vi "Interface.vi"() -> ()   [LabVIEW 2016, in "Program Interface.lvclass"]
uses:
  Program Interface.lvclass
  Universal Robot/Universal Robot.lvclass
  C:/_Code/Development/UR LabVIEW Interface/Classes/Application Interface/Application Interface.lvclass
  Universal Robot/ProgramControlEvent.ctl
  Program Interface.lvclass/Program Interface.ctl
  Application/Application.lvclass
  Application Interface/Application Interface.lvclass
panel:
  out "loadedProgram":string
  out "programStatus":string
  out "programStatusColor":u32(colorbox)
  in  "play":bool
  in  "pause":bool
  in  "stop":bool
  out "returnStatus":string
  in  "load":bool
  in  "programList":i32(listbox)
  in  "addProgram":string
  in  "add program":bool
  in  "play queue":bool
  in  "programQueue":i32(listbox)
  in  "clear queue":bool
  in  "interface":refnum<class "Program Interface.lvclass">
  in  "robot":refnum<class "Universal Robot.lvclass">
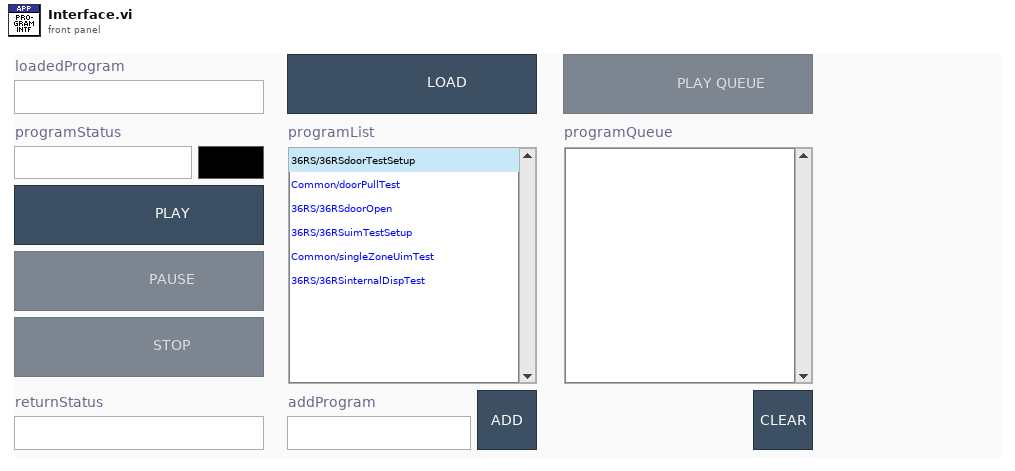
[diagram p1: front panel]
types:
  T1 = typedef "Universal Robot.lvclass/ProgramControlEvent.ctl" = enum16{"Stop", "Pause"}
  T2 = typedef "Application.lvclass/FrontPanelControls.ctl" = cluster{"General Interface":refnum<vi>, "Program Interface":refnum<vi>, "Command Interface":refnum<vi>}
  T3 = typedef "Universal Robot.lvclass/RobotStatus.ctl" = cluster{"Robot Mode":T4, "Operational Mode":T5, "Safety Status":T6, "Remote Control":bool}
  T4 = typedef "Universal Robot.lvclass/RobotMode.ctl" = enum16{"INVALID", "NO_CONTROLLER", "DISCONNECTED", "CONFIRM_SAFETY", "BOOTING", "POWER_OFF", "POWER_ON", "IDLE", "BACKDRIVE", "RUNNING"}
  T5 = typedef "Universal Robot.lvclass/OperationalMode.ctl" = enum16{"NONE", "MANUAL", "AUTOMATIC"}
  T6 = typedef "Universal Robot.lvclass/SafetyStatus.ctl" = enum16{"INVALID", "NORMAL", "REDUCED", "PROTECTIVE_STOP", "RECOVERY", "SAFEGAURD_STOP", "SYSTEM_EMERGENCY_STOP", "ROBOT_EMERGENCY_STOP", "VIOLATION", "FAULT", "AUTOMATIC_MODE_SAFEGAURD_STOP", "SYSTEM_THREE_POSITION_ENABLING_STOP"}
  T7 = typedef "Universal Robot.lvclass/ProgramStatus.ctl" = cluster{"Loaded Program":string, "Valid Program":bool, "Program State":T8, "Running":bool}
  T8 = typedef "Universal Robot.lvclass/ProgramState.ctl" = enum16{"STOPPED", "PLAYING", "PAUSE"}
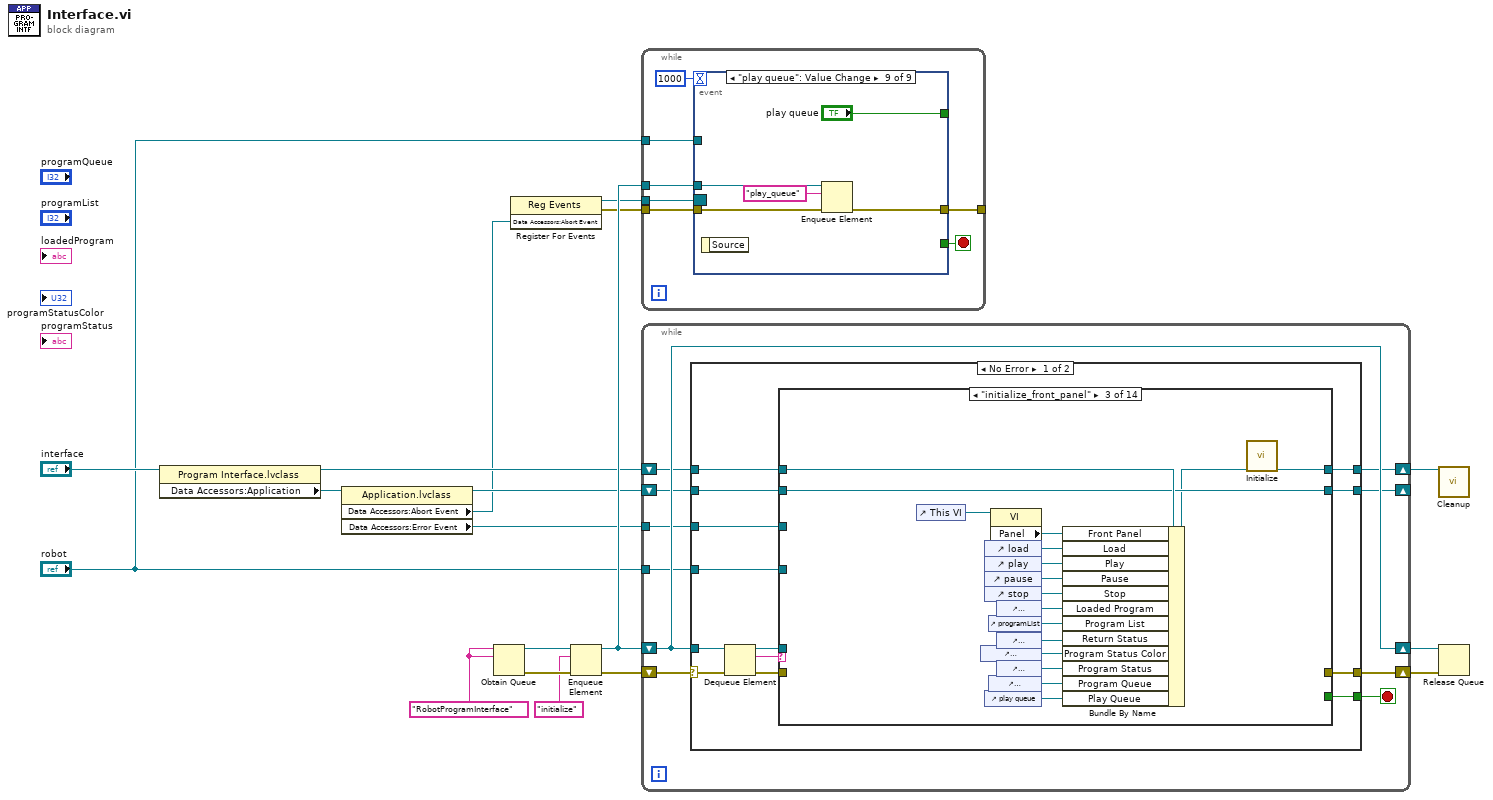
[diagram p0: block diagram]
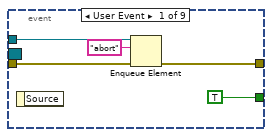
[diagram p2: hidden frame]
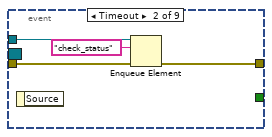
[diagram p3: hidden frame]
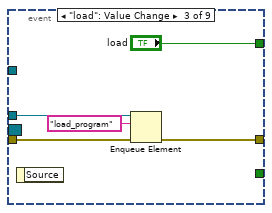
[diagram p4: hidden frame]
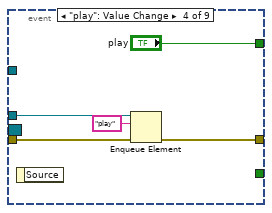
[diagram p5: hidden frame]
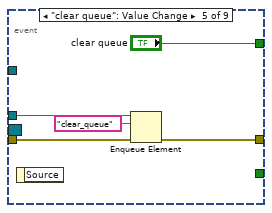
[diagram p6: hidden frame]
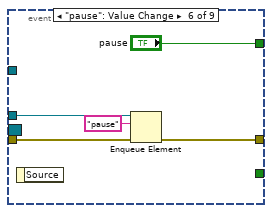
[diagram p7: hidden frame]
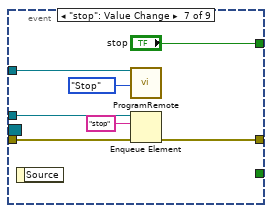
[diagram p8: hidden frame]
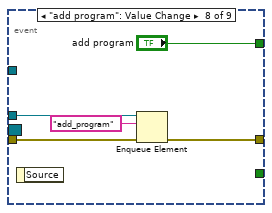
[diagram p9: hidden frame]
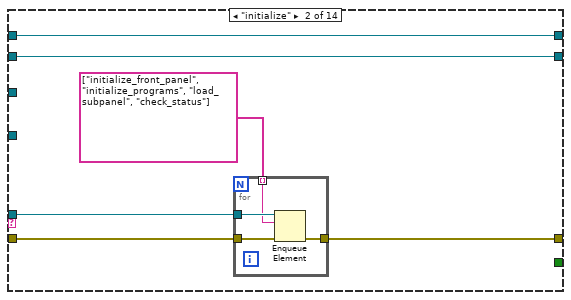
[diagram p11: hidden frame]
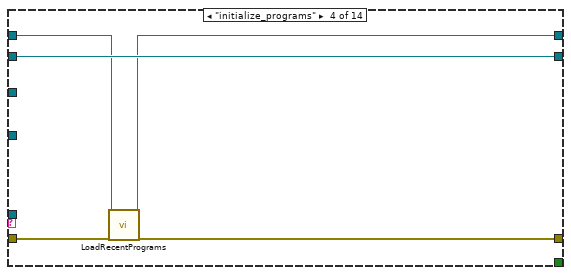
[diagram p12: hidden frame]
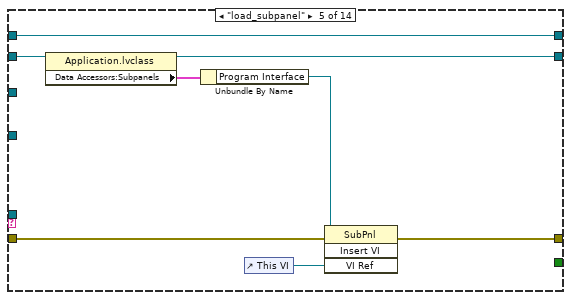
[diagram p13: hidden frame]
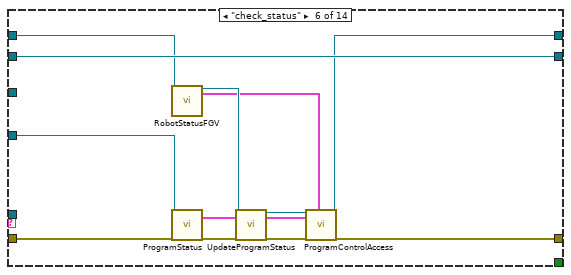
[diagram p14: hidden frame]
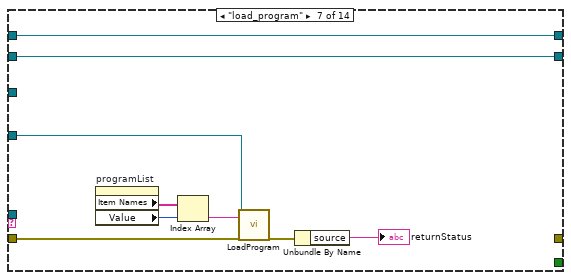
[diagram p15: hidden frame]
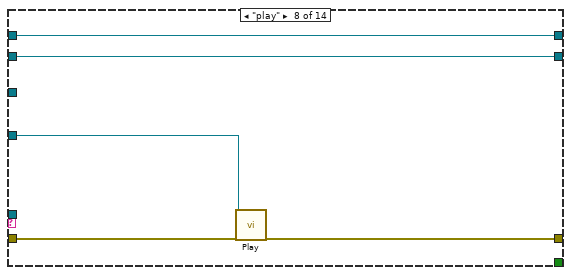
[diagram p16: hidden frame]
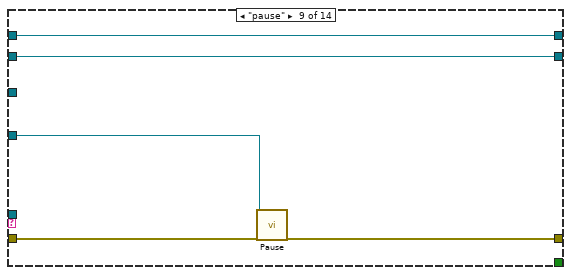
[diagram p17: hidden frame]
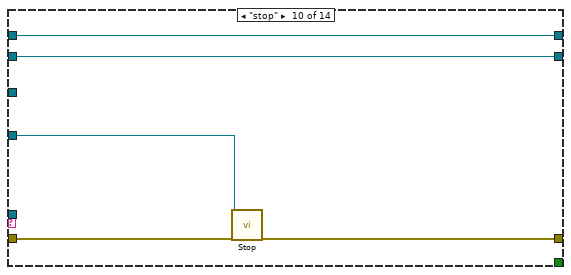
[diagram p18: hidden frame]
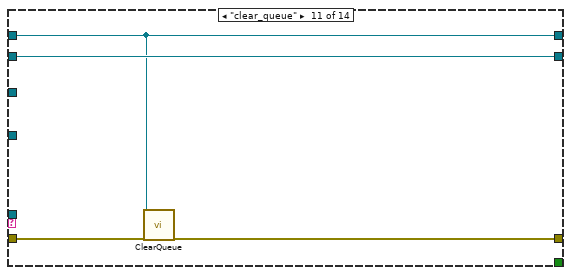
[diagram p19: hidden frame]
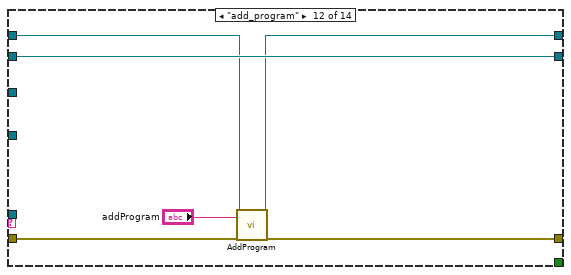
[diagram p20: hidden frame]
diagram:
  w13 = "RobotProgramInterface" ("name (unnamed)")
  n1 = property class="Program Interface.lvclass"(reference="interface") -> (reference out=w5:refnum<class "Program Interface.lvclass">, "Data Accessors:Application"=w8:refnum<class "Application.lvclass">)  [unwired: 1 in, 1 out]
  n2 = property class="Application.lvclass"(reference=w8) -> (reference out=w7:refnum<class "Application.lvclass">, "Data Accessors:Abort Event"=w2:refnum<user-event>, "Data Accessors:Error Event"=w6:refnum<user-event>)  [unwired: 1 in, 1 out]
  n3 = Obtain Queue(name (unnamed)=w13, element data type=w13) -> (queue out=w17:refnum<queue>, error out=w18:errorcluster)  [unwired: 3 in, 1 out]
  n4 = register-events(w2) -> (reference out=w9:refnum<event-registration>, error out=w10:errorcluster)  [unwired: 2 in]
  n5 = Enqueue Element(queue=w17, element="initialize", error in (no error)=w18) -> (queue out=w14:refnum<queue>, error out=w15:errorcluster)  [unwired: 1 in, 1 out]
  n6 = while {
    tunnel: w14 -> [w25]
    tunnel: w10 -> [w24]
    tunnel: w9 -> [w23]
    tunnel: [w22] -> _
    tunnel: "robot" -> [w19]
    stop <- w21 stop-if-true
    n7 = event shown="[8] \"play queue\": Value Change" {
      selector: w23 -> [_ _ _ _ _ _ _ _ _]
      dyn-events: _ -> [_ _ _ _ _ _ _ _ _]
      timeout: 1000 -> [_ _ _ _ _ _ _ _ _]
      tunnel: w25 -> [w30 w34 w39 w44 w49 w54 w61 w66 w71]
      tunnel: w24 -> [w29 w33 w38 w43 w48 w53 w60 w65 w70]
      tunnel: [w28 w32 w37 w42 w47 w52 w59 w64 w69] -> w22
      tunnel: [TRUE _ _ _ _ _ _ _ _] -> w21
      tunnel: [_ _ "load" "play" "clear queue" "pause" "stop" "add program" "play queue"] -> _
      tunnel: w19 -> [_ _ _ _ _ _ w56 _ _]
      event User Event {
        n8 = event-data() -> ()  [unwired: 1 in, 1 out]
        n9 = Enqueue Element(queue=w30, element="abort", error in (no error)=w29) -> (error out=w28:errorcluster)  [unwired: 1 in, 2 out]
      }
      event Timeout {
        n10 = event-data() -> ()  [unwired: 1 in, 1 out]
        n11 = Enqueue Element(queue=w34, element="check_status", error in (no error)=w33) -> (error out=w32:errorcluster)  [unwired: 1 in, 2 out]
      }
      event "load": Value Change {
        n12 = event-data() -> ()  [unwired: 1 in, 1 out]
        n13 = Enqueue Element(queue=w39, element="load_program", error in (no error)=w38) -> (error out=w37:errorcluster)  [unwired: 1 in, 2 out]
      }
      event "play": Value Change {
        n14 = event-data() -> ()  [unwired: 1 in, 1 out]
        n15 = Enqueue Element(queue=w44, element="play", error in (no error)=w43) -> (error out=w42:errorcluster)  [unwired: 1 in, 2 out]
      }
      event "clear queue": Value Change {
        n16 = event-data() -> ()  [unwired: 1 in, 1 out]
        n17 = Enqueue Element(queue=w49, element="clear_queue", error in (no error)=w48) -> (error out=w47:errorcluster)  [unwired: 1 in, 2 out]
      }
      event "pause": Value Change {
        n18 = event-data() -> ()  [unwired: 1 in, 1 out]
        n19 = Enqueue Element(queue=w54, element="pause", error in (no error)=w53) -> (error out=w52:errorcluster)  [unwired: 1 in, 2 out]
      }
      event "stop": Value Change {
        n20 = event-data() -> ()  [unwired: 1 in, 1 out]
        n21 = call-dynamic "ProgramRemote.vi"("Universal Robot.lvclass in"=w56, "Remote"=ProgramControlEvent."Stop") -> ()  [unwired: 16 in, 2 out]
        n22 = Enqueue Element(queue=w61, element="stop", error in (no error)=w60) -> (error out=w59:errorcluster)  [unwired: 1 in, 2 out]
      }
      event "add program": Value Change {
        n23 = event-data() -> ()  [unwired: 1 in, 1 out]
        n24 = Enqueue Element(queue=w66, element="add_program", error in (no error)=w65) -> (error out=w64:errorcluster)  [unwired: 1 in, 2 out]
      }
      event "play queue": Value Change {
        n25 = event-data() -> ()  [unwired: 1 in, 1 out]
        n26 = Enqueue Element(queue=w71, element="play_queue", error in (no error)=w70) -> (error out=w69:errorcluster)  [unwired: 1 in, 2 out]
      }
    }
  }
  n27 = while {
    shift-right: [w79] -> w11
    shift-left: w15 -> [w81]
    shift-right: [w80] -> w12
    shift-left: w14 -> [w80]
    tunnel: "robot" -> [w76]
    tunnel: w6 -> [w75]
    shift-right: [w74] -> _
    shift-left: w7 -> [w77]
    shift-right: [w72] -> w3
    shift-left: w5 -> [w73]
    stop <- w78 stop-if-true
    n28 = case shown="No Error" w81 {
      selector: w81 -> [w93 w202]
      tunnel: w80 -> [w94 _]
      tunnel: [w89 _] -> w79
      tunnel: [w88 _] -> w78
      tunnel: w77 -> [w87 w200]
      tunnel: w76 -> [w86 _]
      tunnel: w75 -> [w85 w203]
      tunnel: [w84 w200] -> w74
      tunnel: w73 -> [w83 w199]
      tunnel: [w82 w199] -> w72
      frame No Error {
        n29 = Dequeue Element(queue=w94, error in (no error)=w93) -> (queue out=w90:refnum<queue>, element=w91:string, error out=w92:errorcluster)  [unwired: 1 in, 1 out]
        n30 = case shown="\"initialize_front_panel\"" w91 {
          tunnel: w92 -> [w97 w99 _ w126 w134 w147 w157 w162 w167 w172 w177 w183 w189 w197]
          tunnel: w90 -> [_ w100 _ _ _ _ _ _ _ _ _ _ _ _]
          tunnel: [w97 w98 _ w125 w137 w148 _ w161 w166 w170 w176 w182 w188 w196] -> w89
          tunnel: [_ _ _ _ _ _ _ _ _ _ _ _ _ TRUE] -> w88
          tunnel: w87 -> [w96 w103 w115 w129 w133 w150 w158 w164 w169 w174 w178 w184 w190 w193]
          tunnel: w86 -> [_ _ _ _ _ w146 w156 w160 w165 w171 _ _ w185 _]
          tunnel: w85 -> [_ _ _ _ _ _ _ _ _ _ _ _ _ _]
          tunnel: [w96 w103 w115 w129 w132 w150 w158 w164 w169 w174 w178 w184 w190 w192] -> w84
          tunnel: w83 -> [w95 w102 w124 w128 w135 w143 w159 w163 w168 w173 w175 w181 w187 w195]
          tunnel: [w95 w102 w110 w127 w135 w149 w159 w163 w168 w173 w175 w180 w186 w195] -> w82
          frame Default {
          }
          frame "initialize" {
            n31 = for {
              tunnel: w100 -> [w107]
              tunnel: w99 -> [w106]
              tunnel: [w105] -> w98
              tunnel: string[] ["initialize_front_panel", "initialize_programs", "load_subpanel", "check_status"] -> [w104] mode=indexing
              n32 = Enqueue Element(queue=w107, element=w104, error in (no error)=w106) -> (error out=w105:errorcluster)  [unwired: 1 in, 2 out]
            }
          }
          frame "initialize_front_panel" {
            n33 = control-ref of="This VI"() -> (w123:refnum<vi>)
            n34 = control-ref of="programStatusColor"() -> (w114:refnum<vi>)
            n35 = control-ref of="load"() -> (w121:refnum<vi>)
            n36 = control-ref of="play"() -> (w120:refnum<vi>)
            n37 = control-ref of="pause"() -> (w119:refnum<vi>)
            n38 = control-ref of="stop"() -> (w118:refnum<vi>)
            n39 = control-ref of="play queue"() -> (w109:refnum<vi>)
            n40 = control-ref of="programList"() -> (w108:refnum<vi>)
            n41 = control-ref of="programQueue"() -> (w112:refnum<vi>)
            n42 = property class="VI"(reference=w123) -> ("Panel"=w122:refnum<vi>)  [unwired: 1 in, 2 out]
            n43 = control-ref of="loadedProgram"() -> (w117:refnum<vi>)
            n44 = control-ref of="returnStatus"() -> (w116:refnum<vi>)
            n45 = control-ref of="programStatus"() -> (w113:refnum<vi>)
            n46 = Bundle By Name(cluster=w124, "Front Panel"=w122, "Load"=w121, "Play"=w120, "Pause"=w119, "Stop"=w118, "Loaded Program"=w117, "Program List"=w108, "Return Status"=w116, "Program Status Color"=w114, "Program Status"=w113, "Program Queue"=w112, "Play Queue"=w109) -> (w111:refnum<class "Program Interface.lvclass">)
            n47 = call "Initialize.vi"("Operation Interface in"=w111) -> ("Operation Interface out"=w110:refnum<class "Program Interface.lvclass">)  [unwired: 18 in]
          }
          frame "initialize_programs" {
            n48 = call "LoadRecentPrograms.vi"("Program Interface in"=w128, "error in (no error)"=w126) -> ("Program Interface out"=w127:refnum<class "Program Interface.lvclass">, "error out"=w125:errorcluster)  [unwired: 16 in]
          }
          frame "load_subpanel" {
            n49 = property class="Application.lvclass"(reference=w133) -> (reference out=w132:refnum<class "Application.lvclass">, "Data Accessors:Subpanels"=w131:T2)  [unwired: 1 in, 1 out]
            n50 = Unbundle By Name(w131) -> ("Program Interface"=w130:refnum<vi>)
            n51 = control-ref of="This VI"() -> (w136:refnum<vi>)
            n52 = invoke class="SubPnl" method="Insert VI"(reference=w130, error in=w134, "VI Ref"=w136) -> (error out=w137:errorcluster)  [unwired: 1 in, 3 out]
          }
          frame "check_status" {
            n53 = call "RobotStatusFGV.vi"("Application Interface in"=w143) -> ("Application Interface out"=w142:refnum<class "Program Interface.lvclass">, "Robot Status out"=w139:T3)  [unwired: 16 in, 1 out]
            n54 = call-dynamic "ProgramStatus.vi"("Universal Robot.lvclass in"=w146, "error in (no error)"=w147) -> ("Program Status"=w145:T7, "error out"=w144:errorcluster)  [unwired: 15 in, 1 out]
            n55 = call "UpdateProgramStatus.vi"("Program Interface in"=w142, "Program Status in"=w145, "error in (no error)"=w144) -> ("Program Interface out"=w141:refnum<class "Program Interface.lvclass">, "Program Status out"=w138:T7, "error out"=w140:errorcluster)  [unwired: 14 in]
            n56 = call "ProgramControlAccess.vi"("Program Interface in"=w141, "Program Status"=w138, "error in (no error)"=w140, "Robot Status"=w139) -> ("Program Interface out"=w149:refnum<class "Program Interface.lvclass">, "error out"=w148:errorcluster)  [unwired: 14 in]
          }
          frame "load_program" {
            n57 = property on="programList" class="LstBox (strict)"() -> ("Item Names"=w155:string[], "Value"=w154:i32)  [unwired: 2 in, 2 out]
            n58 = Index Array(array=w155, index=w154) -> (element=w153:string)
            n59 = call-dynamic "LoadProgram.vi"("Universal Robot.lvclass in"=w156, "program"=w153, "error in (no error)"=w157) -> ("error out"=w152:errorcluster)  [unwired: 15 in, 1 out]
            n60 = Unbundle By Name(w152) -> ("source"=→"returnStatus":string)
          }
          frame "play" {
            n61 = call-dynamic "Play.vi"("Universal Robot.lvclass in"=w160, "error in (no error)"=w162) -> ("error out"=w161:errorcluster)  [unwired: 16 in, 1 out]
          }
          frame "pause" {
            n62 = call-dynamic "Pause.vi"("Universal Robot.lvclass in"=w165, "error in (no error)"=w167) -> ("error out"=w166:errorcluster)  [unwired: 16 in, 1 out]
          }
          frame "stop" {
            n63 = call-dynamic "Stop.vi"("Universal Robot.lvclass in"=w171, "error in (no error)"=w172) -> ("error out"=w170:errorcluster)  [unwired: 16 in, 1 out]
          }
          frame "clear_queue" {
            n64 = call "ClearQueue.vi"("Program Interface in"=w175, "error in (no error)"=w177) -> ("error out"=w176:errorcluster)  [unwired: 16 in, 1 out]
          }
          frame "add_program" {
            n65 = call "AddProgram.vi"("Program Interface in"=w181, "addProgram"="addProgram", "error in (no error)"=w183) -> ("Program Interface out"=w180:refnum<class "Program Interface.lvclass">, "error out"=w182:errorcluster)  [unwired: 15 in]
          }
          frame "play_queue" {
            n66 = call "PlayQueue.vi"("Program Interface in"=w187, "robot"=w185, "error in (no error)"=w189) -> ("Program Interface out"=w186:refnum<class "Program Interface.lvclass">, "error out"=w188:errorcluster)  [unwired: 15 in]
          }
          frame "abort" {
            n67 = property class="Application.lvclass"(reference=w193) -> (reference out=w192:refnum<class "Application.lvclass">, "Data Accessors:Subpanels"=w194:T2)  [unwired: 1 in, 1 out]
            n68 = Unbundle By Name(w194) -> ("Program Interface"=w191:refnum<vi>)
            n69 = invoke class="SubPnl" method="Remove VI"(reference=w191, error in=w197) -> (error out=w196:errorcluster)  [unwired: 1 in, 2 out]
          }
        }
      }
      frame Error {
        n70 = Generate User Event(user event=w203, event data cluster=w202) -> (error out=w201:errorcluster)  [unwired: 2 in, 1 out]
        n71 = call <vilib>:"Clear Errors.vi"("error in (no error)"=w201) -> ()  [unwired: 5 in, 2 out]
      }
    }
  }
  n72 = call "Cleanup.vi"("Operation Interface in"=w3) -> ()  [unwired: 19 in]
  n73 = Release Queue(queue=w12, error in (no error)=w11) -> ()  [unwired: 1 in, 3 out]
